vi "Temperature Monitor.vi"() -> ()   [LabVIEW 2015]
doc: "This VI is the solution to an exercise in the LabVIEW Core 1 course.\n\nIt uses a While Loop and shift registers to average data. No hardware is necessary."
panel:
  out "Œrednia":dbl
  in  "Stop Button":bool
  out "Temperature History":dbl(graph)
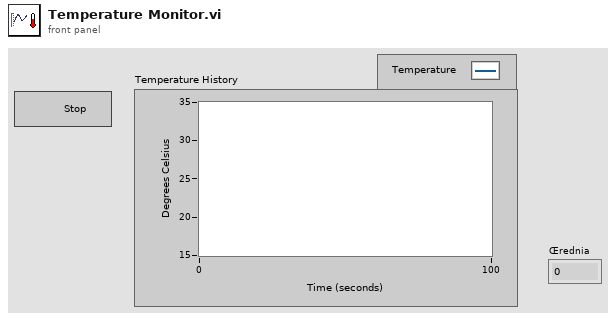
[diagram p1: front panel]
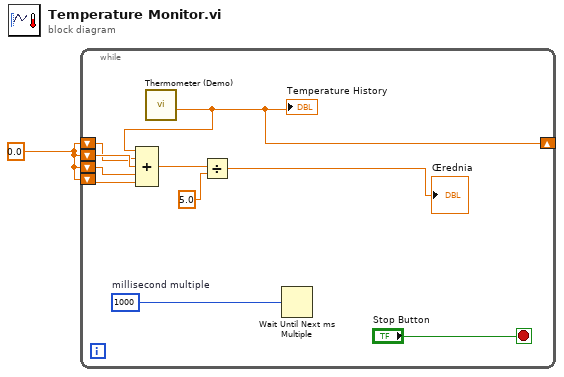
[diagram p0: block diagram]
diagram:
  w1 = 0.0
  n1 = while {
    shift-right: [w7] -> _
    shift-left: w1 -> [w3]
    shift-left: w1 -> [w4]
    shift-left: w1 -> [w6]
    shift-left: w1 -> [w5]
    stop <- "Stop Button" stop-if-true
    w10 = u32 1000  # millisecond multiple
    n2 = call "Thermometer (Demo).vi"() -> ("Temperature Value"=w7:dbl)  [unwired: 11 in]
    "Temperature History" <- w7
    n3 = Compound Arithmetic op=ADD(w7, w3, w4, w6, w5) -> (w2:dbl)
    n4 = Divide(x=w2, y=5.0) -> (x/y=→"Œrednia":dbl)
    n5 = Wait Until Next ms Multiple(millisecond multiple=w10) -> ()  [unwired: 1 out]
  }
